vi "Binary Generate User.vi"   [LabVIEW 2020]
uses:
  [Data] Userinfo/[Data] Abstruct Userinfo/Control/user info.ctl
  [Data] Userinfo/[Data] Userinfo Binary/[Data] Userinfo Binary.lvclass
  <vilib>/YU/YU-Encrypt/MD5/MD5.lvclass
  [Data] Userinfo/[Data] Abstruct Userinfo/[Data] Abstruct Userinfo.lvclass
types:
  T1 = typedef "[Data] Abstruct Userinfo.lvclass/user info.ctl" = cluster{"username":string, "password":string, "authority":i8, "department":string, "post":string, "remark":string, "create time":timestamp, "last login time":timestamp}
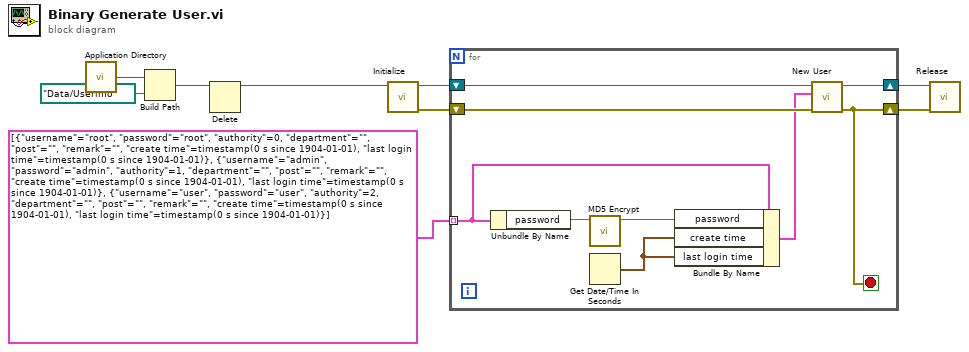
[diagram p0: block diagram]
diagram:
  n1 = call <vilib>:"Application Directory.vi"() -> ("Application Directory"=w9:path)
  n2 = Build Path(base path=w9, name or relative path=path "Data/Userinfo") -> (appended path=w2:path)
  n3 = Delete(path (use dialog)=w2) -> (deleted path=w1:path)  [unwired: 4 in, 2 out]
  n4 = call "Initialize.vi"("userinfo file"=w1) -> ("error out"=w6:errorcluster, "[Data] Userinfo Binary out"=w7:refnum<class "[Data] Userinfo Binary.lvclass">)  [unwired: 9 in]
  n5 = for {
    tunnel: T1[] [{"username"="root", "password"="root", "authority"=0, "department"="", "post"="", "remark"="", "create time"=timestamp(0 s since 1904-01-01), "last login time"=timestamp(0 s since 1904-01-01)}, {"username"="admin", "password"="admin", "authority"=1, "department"="", "post"="", "remark"="", "create time"=timestamp(0 s since 1904-01-01), "last login time"=timestamp(0 s since 1904-01-01)}, {"username"="user", "password"="user", "authority"=2, "department"="", "post"="", "remark"="", "create time"=timestamp(0 s since 1904-01-01), "last login time"=timestamp(0 s since 1904-01-01)}] ("Array") -> [w13] mode=indexing
    shift-right: [w16] -> w3
    shift-left: w7 -> [w18]
    shift-right: [w12] -> w4
    shift-left: w6 -> [w17]
    stop <- w12 stop-if-true
    n6 = Unbundle By Name(w13) -> ("password"=w15:string)
    n7 = call <vilib>:"MD5 Encrypt.vi"("data"=w15) -> ("encrypted data"=w14:string)  [unwired: 9 in, 1 out]
    n8 = Get Date/Time In Seconds() -> (seconds since 1Jan1904=w11:timestamp)
    n9 = Bundle By Name(cluster=w13, "password"=w14, "create time"=w11, "last login time"=w11) -> (w10:T1)
    n10 = call-dynamic "New User.vi"("error in (no error)"=w17, "user info"=w10, "[Data] Userinfo Binary in"=w18) -> ("error out"=w12:errorcluster, "[Data] Userinfo Binary out"=w16:refnum<class "[Data] Userinfo Binary.lvclass">)  [unwired: 7 in]
  }
  n11 = call "Release.vi"("error in (no error)"=w4, "[Data] Userinfo Binary in"=w3) -> ()  [unwired: 8 in, 2 out]
